vi "DAQmx Create Channel (AO-FuncGen).vi"(0 "task in":refnum<k21>, 1 "frequency":dbl=1000.0 format="%.2f", 2 "amplitude":dbl=5.0 format="%.2f", 3 "offset":dbl format="%.2f", 5 "physical channels":tag, 7 "name to assign":string, 9 "type":i32(ring)=14751 items=["Sine"=14751, "Triangle"=14752, "Square"=14753, "Sawtooth"=14754], 11 "error in":errorcluster) -> (4 "task out":refnum<k21>, 15 "error out":errorcluster)   [LabVIEW 2013]
doc: "Creates a channel for continually generating a waveform on the selected physical channel."
uses:
  C:/Program Files/National Instruments/LabVIEW 2013/resource/objmgr/daqmx.rc
panel:
  # "output limits"
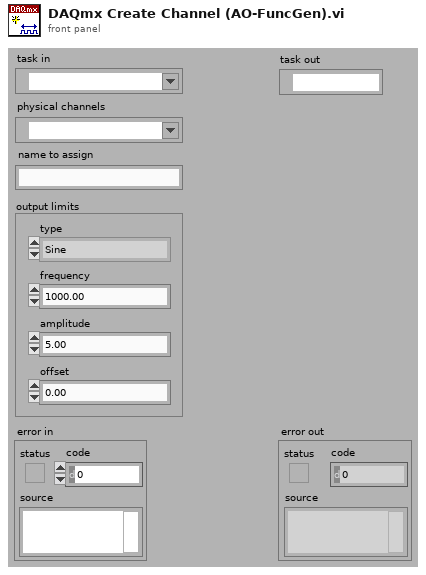
[diagram p1: front panel]
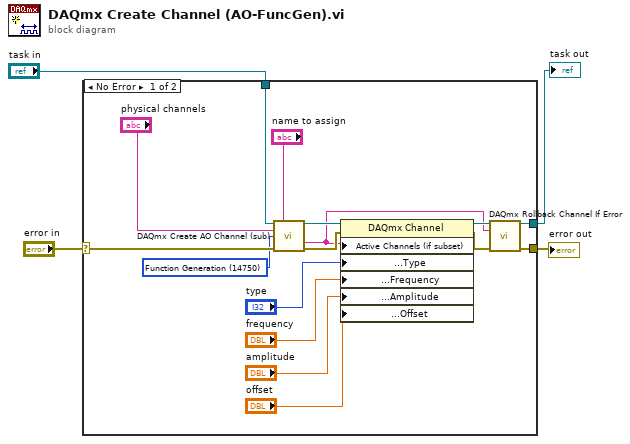
[diagram p0: block diagram]
diagram:
  n1 = case shown="No Error" "error in" {
    selector: "error in" -> [w18 w22]
    tunnel: [w14 w22] -> w4
    tunnel: "task in" -> [w20 w21]
    tunnel: [w12 w21] -> w1
    frame No Error {
      w9 = 14750 items=["Voltage"=10322, "Current"=10134, "Function Generation"=14750] ("AO.OutputType")
      n2 = call "DAQmx Create AO Channel (sub).vi"("task in"=w20, "virtual channel name"="name to assign", "physical channel name"="physical channels", "output type"=w9, "error in"=w18) -> ("task out"=w15:refnum<k21>, "channel names"=w10:string, "error out"=w17:errorcluster)  [unwired: 2 in, 6 out]
      n3 = property class="DAQmx Channel"(reference=w15, error in=w17, "Active Channels (if subset)"=w10, "Analog Output:Function Generation:Type"="type", "Analog Output:Function Generation:Frequency"="frequency", "Analog Output:Function Generation:Amplitude"="amplitude", "Analog Output:Function Generation:Offset"="offset") -> (reference out=w13:refnum<k21>, error out=w11:errorcluster)
      n4 = call "DAQmx Rollback Channel If Error.vi"("task in"=w13, "channel names"=w10, "error in"=w11) -> ("task out"=w12:refnum<k21>, "error out"=w14:errorcluster)  [unwired: 11 out]
    }
    frame Error {
    }
  }
  "error out" <- w4
  "task out" <- w1
